vi "GeoData.vi"() -> ()   [LabVIEW 2017] (continued)
Brandywine\tMD\tCharles County\tH1\n20616\t24017\tBryans road\tMD\tCharles County\tH1\n21613\t24019\tCambridge\tMD\tDorchester County\tH1\n21648\t24019\tMadison\tMD\tDorchester County\tH1\n21626\t24019\tCrapo\tMD\tDorchester County\tH1\n21675\t24019\tWingate\tMD\tDorchester County\tH1\n21669\t24019\tTaylors island\tMD\tDorchester County\tH1\n21655\t24019\tPreston\tMD\tDorchester County\tH1\n21664\t24019\tSecretary\tMD\tDorchester County\tH1\n21835\t24019\tLinkwood\tMD\tDorchester County\tH1\n21672\t24019\tToddville\tMD\tDorchester County\tH1\n21622\t24019\tChurch creek\tMD\tDorchester County\tH1\n21631\t24019\tEast new market\tMD\tDorchester County\tH1\n21659\t24019\tRhodesdale\tMD\tDorchester County\tH1\n21632\t24019\tFederalsburg\tMD\tDorchester County\tH1\n21643\t24019\tHurlock\tMD\tDorchester County\tH1\n21677\t24019\tWoolford\tMD\tDorchester County\tH1\n21627\t24019\tCrocheron\tMD\tDorchester County\tH1\n21869\t24019\tVienna\tMD\tDorchester County\tH1\n21634\t24019\tFishing creek\tMD\tDorchester County\tH1\n20842\t24021\tDickerson\tMD\tFrederick County\tH1\n21757\t24021\tKeymar\tMD\tFrederick County\tH1\n21783\t24021\tSmithsburg\tMD\tFrederick County\tH1\n21719\t24021\tCascade\tMD\tFrederick County\tH1\n21759\t24021\tLadiesburg\tMD\tFrederick County\tH1\n21704\t24021\tFrederick\tMD\tFrederick County\tH1\n21771\t24021\tMount airy\tMD\tFrederick County\tH1\n21773\t24021\tMyersville\tMD\tFrederick County\tH1\n21787\t24021\tTaneytown\tMD\tFrederick County\tH1\n21793\t24021\tWalkersville\tMD\tFrederick County\tH1\n21798\t24021\tWoodsboro\tMD\tFrederick County\tH1\n21790\t24021\tTuscarora\tMD\tFrederick County\tH1\n20871\t24021\tClarksburg\tMD\tFrederick County\tH1\n21774\t24021\tNew market\tMD\tFrederick County\tH1\n21727\t24021\tEmmitsburg\tMD\tFrederick County\tH1\n21769\t24021\tMiddletown\tMD\tFrederick County\tH1\n21780\t24021\tSabillasville\tMD\tFrederick County\tH1\n21714\t24021\tBraddock heights\tMD\tFrederick County\tH1\n21703\t24021\tFrederick\tMD\tFrederick County\tH1\n21770\t24021\tMonrovia\tMD\tFrederick County\tH1\n21754\t24021\tIjamsville\tMD\tFrederick County\tH1\n21755\t24021\tJefferson\tMD\tFrederick County\tH1\n21717\t24021\tBuckeystown\tMD\tFrederick County\tH1\n21778\t24021\tRocky ridge\tMD\tFrederick County\tH1\n21776\t24021\tNew windsor\tMD\tFrederick County\tH1\n21791\t24021\tUnion bridge\tMD\tFrederick County\tH1\n21762\t24021\tLibertytown\tMD\tFrederick County\tH1\n21716\t24021\tBrunswick\tMD\tFrederick County\tH1\n21710\t24021\tAdamstown\tMD\tFrederick County\tH1\n21758\t24021\tKnoxville\tMD\tFrederick County\tH1\n21777\t24021\tPoint of rocks\tMD\tFrederick County\tH1\n21775\t24021\tNew midway\tMD\tFrederick County\tH1\n21701\t24021\tFrederick\tMD\tFrederick County\tH1\n21702\t24021\tFrederick\tMD\tFrederick County\tH1\n21713\t24021\tBoonsboro\tMD\tFrederick County\tH1\n21705\t24021\tFrederick\tMD\tFrederick County\tH1\n21788\t24021\tThurmont\tMD\tFrederick County\tH1\n21718\t24021\tBurkittsville\tMD\tFrederick County\tH1\n21531\t24023\tFriendsville\tMD\tGarrett County\tH1\n21538\t24023\tKitzmiller\tMD\tGarrett County\tH1\n21562\t24023\tWesternport\tMD\tGarrett County\tH1\n21536\t24023\tGrantsville\tMD\tGarrett County\tH1\n21521\t24023\tBarton\tMD\tGarrett County\tH1\n21523\t24023\tBloomington\tMD\tGarrett County\tH1\n21532\t24023\tFrostburg\tMD\tGarrett County\tH1\n21541\t24023\tMc henry\tMD\tGarrett County\tH1\n21561\t24023\tSwanton\tMD\tGarrett County\tH1\n21522\t24023\tBittinger\tMD\tGarrett County\tH1\n21539\t24023\tLonaconing\tMD\tGarrett County\tH1\n21520\t24023\tAccident\tMD\tGarrett County\tH1\n21550\t24023\tOakland\tMD\tGarrett County\tH1\n21014\t24025\tBel air\tMD\tHarford County\tH1\n21034\t24025\tDarlington\tMD\tHarford County\tH1\n21050\t24025\tForest hill\tMD\tHarford County\tH1\n21087\t24025\tKingsville\tMD\tHarford County\tH1\n21160\t24025\tWhiteford\tMD\tHarford County\tH1\n21154\t24025\tStreet\tMD\tHarford County\tH1\n21010\t24025\tGunpowder\tMD\tHarford County\tH1\n21047\t24025\tFallston\tMD\tHarford County\tH1\n21084\t24025\tJarrettsville\tMD\tHarford County\tH1\n21078\t24025\tHavre de grace\tMD\tHarford County\tH1\n21018\t24025\tBenson\tMD\tHarford County\tH1\n21001\t24025\tAberdeen\tMD\tHarford County\tH1\n21028\t24025\tChurchville\tMD\tHarford County\tH1\n21085\t24025\tJoppa\tMD\tHarford County\tH1\n21111\t24025\tMonkton\tMD\tHarford County\tH1\n21130\t24025\tPerryman\tMD\tHarford County\tH1\n21005\t24025\tAberdeen proving ground\tMD\tHarford County\tH1\n21082\t24025\tHydes\tMD\tHarford County\tH1\n21132\t24025\tPylesville\tMD\tHarford County\tH1\n21161\t24025\tWhite hall\tMD\tHarford County\tH1\n21017\t24025\tBelcamp\tMD\tHarford County\tH1\n21009\t24025\tAbingdon\tMD\tHarford County\tH1\n21040\t24025\tEdgewood\tMD\tHarford County\tH1\n21015\t24025\tBel air\tMD\tHarford County\tH1\n21013\t24025\tBaldwin\tMD\tHarford County\tH1\n21043\t24027\tEllicott city\tMD\tHoward County\tH1\n21046\t24027\tColumbia\tMD\tHoward County\tH1\n21737\t24027\tGlenelg\tMD\tHoward County\tH1\n20777\t24027\tHighland\tMD\tHoward County\tH1\n21771\t24027\tMount airy\tMD\tHoward County\tH1\n21784\t24027\tSykesville\tMD\tHoward County\tH1\n21738\t24027\tGlenwood\tMD\tHoward County\tH1\n21794\t24027\tWest friendship\tMD\tHoward County\tH1\n20723\t24027\tLaurel\tMD\tHoward County\tH1\n20794\t24027\tJessup\tMD\tHoward County\tH1\n21044\t24027\tColumbia\tMD\tHoward County\tH1\n21041\t24027\tEllicott city\tMD\tHoward County\tH1\n21042\t24027\tEllicott city\tMD\tHoward County\tH1\n21036\t24027\tDayton\tMD\tHoward County\tH1\n21075\t24027\tElkridge\tMD\tHoward County\tH1\n21163\t24027\tWoodstock\tMD\tHoward County\tH1\n21765\t24027\tLisbon\tMD\tHoward County\tH1\n21150\t24027\tSimpsonville\tMD\tHoward County\tH1\n20763\t24027\tSavage\tMD\tHoward County\tH1\n20759\t24027\tFulton\tMD\tHoward County\tH1\n21029\t24027\tClarksville\tMD\tHoward County\tH1\n21076\t24027\tHanover\tMD\tHoward County\tH1\n21723\t24027\tCooksville\tMD\tHoward County\tH1\n20701\t24027\tAnnapolis junction\tMD\tHoward County\tH1\n20833\t24027\tBrookeville\tMD\tHoward County\tH1\n21045\t24027\tColumbia\tMD\tHoward County\tH1\n21797\t24027\tWoodbine\tMD\tHoward County\tH1\n21104\t24027\tMarriottsville\tMD\tHoward County\tH1\n21645\t24029\tKennedyville\tMD\tKent County\tH1\n21667\t24029\tStill pond\tMD\tKent County\tH1\n21610\t24029\tBetterton\tMD\tKent County\tH1\n21635\t24029\tGalena\tMD\tKent County\tH1\n21651\t24029\tMillington\tMD\tKent County\tH1\n21678\t24029\tWorton\tMD\tKent County\tH1\n21690\t24029\tChestertown\tMD\tKent County\tH1\n21930\t24029\tGeorgetown\tMD\tKent County\tH1\n21620\t24029\tChestertown\tMD\tKent County\tH1\n21661\t24029\tRock hall\tMD\tKent County\tH1\n21650\t24029\tMassey\tMD\tKent County\tH1\n20815\t24031\tChevy chase\tMD\tMontgomery County\tH1\n20816\t24031\tBethesda\tMD\tMontgomery County\tH1\n20841\t24031\tBoyds\tMD\tMontgomery County\tH1\n20842\t24031\tDickerson\tMD\tMontgomery County\tH1\n20906\t24031\tSilver spring\tMD\tMontgomery County\tH1\n20777\t24031\tHighland\tMD\tMontgomery County\tH1\n20884\t24031\tGaithersburg\tMD\tMontgomery County\tH1\n20818\t24031\tCabin john\tMD\tMontgomery County\tH1\n20852\t24031\tRockville\tMD\tMontgomery County\tH1\n20914\t24031\tSilver spring\tMD\tMontgomery County\tH1\n20915\t24031\tSilver spring\tMD\tMontgomery County\tH1\n21771\t24031\tMount airy\tMD\tMontgomery County\tH1\n20880\t24031\tWashington grove\tMD\tMontgomery County\tH1\n20918\t24031\tSilver spring\tMD\tMontgomery County\tH1\n20849\t24031\tRockville\tMD\tMontgomery County\tH1\n20911\t24031\tSilver spring\tMD\tMontgomery County\tH1\n20859\t24031\tPotomac\tMD\tMontgomery County\tH1\n20993\t24031\tSilver spring\tMD\tMontgomery County\tH1\n20854\t24031\tPotomac\tMD\tMontgomery County\tH1\n20868\t24031\tSpencerville\tMD\tMontgomery County\tH1\n20871\t24031\tClarksburg\tMD\tMontgomery County\tH1\n20882\t24031\tGaithersburg\tMD\tMontgomery County\tH1\n20838\t24031\tBarnesville\tMD\tMontgomery County\tH1\n20898\t24031\tGaithersburg\tMD\tMontgomery County\tH1\n20830\t24031\tOlney\tMD\tMontgomery County\tH1\n20892\t24031\tBethesda\tMD\tMontgomery County\tH1\n20783\t24031\tHyattsville\tMD\tMontgomery County\tH1\n20832\t24031\tOlney\tMD\tMontgomery County\tH1\n20861\t24031\tAshton\tMD\tMontgomery County\tH1\n20903\t24031\tSilver spring\tMD\tMontgomery County\tH1\n21770\t24031\tMonrovia\tMD\tMontgomery County\tH1\n20862\t24031\tBrinklow\tMD\tMontgomery County\tH1\n20811\t24031\tBethesda\tMD\tMontgomery County\tH1\n20817\t24031\tBethesda\tMD\tMontgomery County\tH1\n20874\t24031\tGermantown\tMD\tMontgomery County\tH1\n20851\t24031\tRockville\tMD\tMontgomery County\tH1\n20860\t24031\tSandy spring\tMD\tMontgomery County\tH1\n20901\t24031\tSilver spring\tMD\tMontgomery County\tH1\n20902\t24031\tSilver spring\tMD\tMontgomery County\tH1\n20899\t24031\tGaithersburg\tMD\tMontgomery County\tH1\n20827\t24031\tBethesda\tMD\tMontgomery County\tH1\n20812\t24031\tGlen echo\tMD\tMontgomery County\tH1\n20847\t24031\tRockville\tMD\tMontgomery County\tH1\n20839\t24031\tBeallsville\tMD\tMontgomery County\tH1\n20857\t24031\tRockville\tMD\tMontgomery County\tH1\n20058\t24031\tWashington\tMD\tMontgomery County\tH1\n20707\t24031\tLaurel\tMD\tMontgomery County\tH1\n20787\t24031\tHyattsville\tMD\tMontgomery County\tH1\n20853\t24031\tRockville\tMD\tMontgomery County\tH1\n20855\t24031\tDerwood\tMD\tMontgomery County\tH1\n20872\t24031\tDamascus\tMD\tMontgomery County\tH1\n20875\t24031\tGermantown\tMD\tMontgomery County\tH1\n20878\t24031\tGaithersburg\tMD\tMontgomery County\tH1\n20886\t24031\tMontgomery village\tMD\tMontgomery County\tH1\n20891\t24031\tKensington\tMD\tMontgomery County\tH1\n20912\t24031\tTakoma park\tMD\tMontgomery County\tH1\n20824\t24031\tBethesda\tMD\tMontgomery County\tH1\n20885\t24031\tGaithersburg\tMD\tMontgomery County\tH1\n20907\t24031\tSilver spring\tMD\tMontgomery County\tH1\n20825\t24031\tChevy chase\tMD\tMontgomery County\tH1\n20883\t24031\tGaithersburg\tMD\tMontgomery County\tH1\n20894\t24031\tBethesda\tMD\tMontgomery County\tH1\n20837\t24031\tPoolesville\tMD\tMontgomery County\tH1\n20904\t24031\tSilver spring\tMD\tMontgomery County\tH1\n20895\t24031\tKensington\tMD\tMontgomery County\tH1\n20879\t24031\tGaithersburg\tMD\tMontgomery County\tH1\n20877\t24031\tGaithersburg\tMD\tMontgomery County\tH1\n20910\t24031\tSilver spring\tMD\tMontgomery County\tH1\n20913\t24031\tTakoma park\tMD\tMontgomery County\tH1\n20848\t24031\tRockville\tMD\tMontgomery County\tH1\n20896\t24031\tGarrett park\tMD\tMontgomery County\tH1\n20889\t24031\tBethesda\tMD\tMontgomery County\tH1\n20916\t24031\tSilver spring\tMD\tMontgomery County\tH1\n20810\t24031\tBethesda\tMD\tMontgomery County\tH1\n20814\t24031\tBethesda\tMD\tMontgomery County\tH1\n20850\t24031\tRockville\tMD\tMontgomery County\tH1\n20833\t24031\tBrookeville\tMD\tMontgomery County\tH1\n20876\t24031\tGermantown\tMD\tMontgomery County\tH1\n20866\t24031\tBurtonsville\tMD\tMontgomery County\tH1\n20905\t24031\tSilver spring\tMD\tMontgomery County\tH1\n21797\t24031\tWoodbine\tMD\tMontgomery County\tH1\n20207\t24031\tWashington\tMD\tMontgomery County\tH1\n20705\t24033\tBeltsville\tMD\tPrince George's County\tH1\n20710\t24033\tBladensburg\tMD\tPrince George's County\tH1\n20721\t24033\tBowie\tMD\tPrince George's County\tH1\n20623\t24033\tCheltenham\tMD\tPrince George's County\tH1\n20718\t24033\tBowie\tMD\tPrince George's County\tH1\n20773\t24033\tUpper marlboro\tMD\tPrince George's County\tH1\n20799\t24033\tCapitol heights\tMD\tPrince George's County\tH1\n20720\t24033\tBowie\tMD\tPrince George's County\tH1\n20715\t24033\tBowie\tMD\tPrince George's County\tH1\n20726\t24033\tLaurel\tMD\tPrince George's County\tH1\n20742\t24033\tCollege park\tMD\tPrince George's County\tH1\n20771\t24033\tGreenbelt\tMD\tPrince George's County\tH1\n20782\t24033\tHyattsville\tMD\tPrince George's County\tH1\n20791\t24033\tCapitol heights\tMD\tPrince George's County\tH1\n20775\t24033\tUpper marlboro\tMD\tPrince George's County\tH1\n20757\t24033\tTemple hills\tMD\tPrince George's County\tH1\n20749\t24033\tFort washington\tMD\tPrince George's County\tH1\n20750\t24033\tOxon hill\tMD\tPrince George's County\tH1\n20389\t24033\tWashington\tMD\tPrince George's County\tH1\n20395\t24033\tWashington\tMD\tPrince George's County\tH1\n20716\t24033\tBowie\tMD\tPrince George's County\tH1\n20724\t24033\tLaurel\tMD\tPrince George's County\tH1\n20745\t24033\tOxon hill\tMD\tPrince George's County\tH1\n20769\t24033\tGlenn dale\tMD\tPrince George's County\tH1\n20772\t24033\tUpper marlboro\tMD\tPrince George's County\tH1\n20783\t24033\tHyattsville\tMD\tPrince George's County\tH1\n20903\t24033\tSilver spring\tMD\tPrince George's County\tH1\n20709\t24033\tLaurel\tMD\tPrince George's County\tH1\n20741\t24033\tCollege park\tMD\tPrince George's County\tH1\n20768\t24033\tGreenbelt\tMD\tPrince George's County\tH1\n20703\t24033\tLanham\tMD\tPrince George's County\tH1\n20731\t24033\tCapitol heights\tMD\tPrince George's County\tH1\n20608\t24033\tAquasco\tMD\tPrince George's County\tH1\n20708\t24033\tLaurel\tMD\tPrince George's County\tH1\n20712\t24033\tMount rainier\tMD\tPrince George's County\tH1\n20740\t24033\tCollege park\tMD\tPrince George's County\tH1\n20792\t24033\tUpper marlboro\tMD\tPrince George's County\tH1\n20753\t24033\tDistrict heights\tMD\tPrince George's County\tH1\n20707\t24033\tLaurel\tMD\tPrince George's County\tH1\n20706\t24033\tLanham\tMD\tPrince George's County\tH1\n20743\t24033\tCapitol heights\tMD\tPrince George's County\tH1\n20737\t24033\tRiverdale\tMD\tPrince George's County\tH1\n20748\t24033\tTemple hills\tMD\tPrince George's County\tH1\n20774\t24033\tUpper marlboro\tMD\tPrince George's County\tH1\n20784\t24033\tHyattsville\tMD\tPrince George's County\tH1\n20912\t24033\tTakoma park\tMD\tPrince George's County\tH1\n20599\t24033\tWashington\tMD\tPrince George's County\tH1\n20601\t24033\tWaldorf\tMD\tPrince George's County\tH1\n20735\t24033\tClinton\tMD\tPrince George's County\tH1\n20746\t24033\tSuitland\tMD\tPrince George's County\tH1\n20781\t24033\tHyattsville\tMD\tPrince George's County\tH1\n20904\t24033\tSilver spring\tMD\tPrince George's County\tH1\n20725\t24033\tLaurel\tMD\tPrince George's County\tH1\n20722\t24033\tBrentwood\tMD\tPrince George's County\tH1\n20704\t24033\tBeltsville\tMD\tPrince George's County\tH1\n20717\t24033\tBowie\tMD\tPrince George's County\tH1\n20588\t24033\tDhs\tMD\tPrince George's County\tH1\n20790\t24033\tCapitol heights\tMD\tPrince George's County\tH1\n20607\t24033\tAccokeek\tMD\tPrince George's County\tH1\n20613\t24033\tBrandywine\tMD\tPrince George's County\tH1\n20616\t24033\tBryans road\tMD\tPrince George's County\tH1\n20744\t24033\tFort washington\tMD\tPrince George's County\tH1\n20770\t24033\tGreenbelt\tMD\tPrince George's County\tH1\n20747\t24033\tDistrict heights\tMD\tPrince George's County\tH1\n20762\t24033\tAndrews air force base\tMD\tPrince George's County\tH1\n20785\t24033\tHyattsville\tMD\tPrince George's County\tH1\n20866\t24033\tBurtonsville\tMD\tPrince George's County\tH1\n20738\t24033\tRiverdale\tMD\tPrince George's County\tH1\n20233\t24033\tWashington\tMD\tPrince George's County\tH1\n20752\t24033\tSuitland\tMD\tPrince George's County\tH1\n21619\t24035\tChester\tMD\tQueen Anne's County\tH1\n21644\t24035\tIngleside\tMD\tQueen Anne's County\tH1\n21679\t24035\tWye mills\tMD\tQueen Anne's County\tH1\n21656\t24035\tPrice\tMD\tQueen Anne's County\tH1\n21651\t24035\tMillington\tMD\tQueen Anne's County\tH1\n21668\t24035\tSudlersville\tMD\tQueen Anne's County\tH1\n21640\t24035\tHenderson\tMD\tQueen Anne's County\tH1\n21649\t24035\tMarydel\tMD\tQueen Anne's County\tH1\n21638\t24035\tGrasonville\tMD\tQueen Anne's County\tH1\n21657\t24035\tQueen anne\tMD\tQueen Anne's County\tH1\n21666\t24035\tStevensville\tMD\tQueen Anne's County\tH1\n21607\t24035\tBarclay\tMD\tQueen Anne's County\tH1\n21623\t24035\tChurch hill\tMD\tQueen Anne's County\tH1\n21628\t24035\tCrumpton\tMD\tQueen Anne's County\tH1\n21670\t24035\tTempleville\tMD\tQueen Anne's County\tH1\n21620\t24035\tChestertown\tMD\tQueen Anne's County\tH1\n21617\t24035\tCentreville\tMD\tQueen Anne's County\tH1\n21658\t24035\tQueenstown\tMD\tQueen Anne's County\tH1\n20634\t24037\tGreat mills\tMD\tSt. Mary's County\tH1\n20692\t24037\tValley lee\tMD\tSt. Mary's County\tH1\n20626\t24037\tColtons point\tMD\tSt. Mary's County\tH1\n20620\t24037\tCallaway\tMD\tSt. Mary's County\tH1\n20670\t24037\tPatuxent river\tMD\tSt. Mary's County\tH1\n20659\t24037\tMechanicsville\tMD\tSt. Mary's County\tH1\n20630\t24037\tDrayden\tMD\tSt. Mary's County\tH1\n20609\t24037\tAvenue\tMD\tSt. Mary's County\tH1\n20628\t24037\tDameron\tMD\tSt. Mary's County\tH1\n20635\t24037\tHelen\tMD\tSt. Mary's County\tH1\n20622\t24037\tCharlotte hall\tMD\tSt. Mary's County\tH1\n20684\t24037\tSaint inigoes\tMD\tSt. Mary's County\tH1\n20618\t24037\tBushwood\tMD\tSt. Mary's County\tH1\n20686\t24037\tSaint marys city\tMD\tSt. Mary's County\tH1\n20619\t24037\tCalifornia\tMD\tSt. Mary's County\tH1\n20653\t24037\tLexington park\tMD\tSt. Mary's County\tH1\n20690\t24037\tTall timbers\tMD\tSt. Mary's County\tH1\n20660\t24037\tMorganza\tMD\tSt. Mary's County\tH1\n20624\t24037\tClements\tMD\tSt. Mary's County\tH1\n20674\t24037\tPiney point\tMD\tSt. Mary's County\tH1\n20680\t24037\tRidge\tMD\tSt. Mary's County\tH1\n20650\t24037\tLeonardtown\tMD\tSt. Mary's County\tH1\n20606\t24037\tAbell\tMD\tSt. Mary's County\tH1\n20656\t24037\tLoveville\tMD\tSt. Mary's County\tH1\n20687\t24037\tScotland\tMD\tSt. Mary's County\tH1\n20621\t24037\tChaptico\tMD\tSt. Mary's County\tH1\n20636\t24037\tHollywood\tMD\tSt. Mary's County\tH1\n20667\t24037\tPark hall\tMD\tSt. Mary's County\tH1\n20627\t24037\tCompton\tMD\tSt. Mary's County\tH1\n21817\t24039\tCrisfield\tMD\tSomerset County\tH1\n21821\t24039\tDeal island\tMD\tSomerset County\tH1\n21838\t24039\tMarion station\tMD\tSomerset County\tH1\n21851\t24039\tPocomoke city\tMD\tSomerset County\tH1\n21857\t24039\tRehobeth\tMD\tSomerset County\tH1\n21836\t24039\tManokin\tMD\tSomerset County\tH1\n21824\t24039\tEwell\tMD\tSomerset County\tH1\n21866\t24039\tTylerton\tMD\tSomerset County\tH1\n21867\t24039\tUpper fairmount\tMD\tSomerset County\tH1\n21871\t24039\tWestover\tMD\tSomerset County\tH1\n21890\t24039\tWestover\tMD\tSomerset County\tH1\n21853\t24039\tPrincess anne\tMD\tSomerset County\tH1\n21822\t24039\tEden\tMD\tSomerset County\tH1\n21601\t24041\tEaston\tMD\tTalbot County\tH1\n21665\t24041\tSherwood\tMD\tTalbot County\tH1\n21679\t24041\tWye mills\tMD\tTalbot County\tH1\n21671\t24041\tTilghman\tMD\tTalbot County\tH1\n21647\t24041\tMcdaniel\tMD\tTalbot County\tH1\n21657\t24041\tQueen anne\tMD\tTalbot County\tH1\n21673\t24041\tTrappe\tMD\tTalbot County\tH1\n21663\t24041\tSaint michaels\tMD\tTalbot County\tH1\n21652\t24041\tNeavitt\tMD\tTalbot County\tH1\n21654\t24041\tOxford\tMD\tTalbot County\tH1\n21624\t24041\tClaiborne\tMD\tTalbot County\tH1\n21662\t24041\tRoyal oak\tMD\tTalbot County\tH1\n21625\t24041\tCordova\tMD\tTalbot County\tH1\n21676\t24041\tWittman\tMD\tTalbot County\tH1\n21612\t24041\tBozman\tMD\tTalbot County\tH1\n21653\t24041\tNewcomb\tMD\tTalbot County\tH1\n21783\t24043\tSmithsburg\tMD\tWashington County\tH1\n21719\t24043\tCascade\tMD\tWashington County\tH1\n21779\t24043\tRohrersville\tMD\tWashington County\tH1\n21721\t24043\tChewsville\tMD\tWashington County\tH1\n21767\t24043\tMaugansville\tMD\tWashington County\tH1\n21746\t24043\tHagerstown\tMD\tWashington County\tH1\n21781\t24043\tSaint james\tMD\tWashington County\tH1\n21769\t24043\tMiddletown\tMD\tWashington County\tH1\n21780\t24043\tSabillasville\tMD\tWashington County\tH1\n21715\t24043\tBrownsville\tMD\tWashington County\tH1\n21740\t24043\tHagerstown\tMD\tWashington County\tH1\n21755\t24043\tJefferson\tMD\tWashington County\tH1\n21720\t24043\tCavetown\tMD\tWashington County\tH1\n21711\t24043\tBig pool\tMD\tWashington County\tH1\n21750\t24043\tHancock\tMD\tWashington County\tH1\n21733\t24043\tFairplay\tMD\tWashington County\tH1\n21758\t24043\tKnoxville\tMD\tWashington County\tH1\n21795\t24043\tWilliamsport\tMD\tWashington County\tH1\n21756\t24043\tKeedysville\tMD\tWashington County\tH1\n21734\t24043\tFunkstown\tMD\tWashington County\tH1\n21713\t24043\tBoonsboro\tMD\tWashington County\tH1\n21742\t24043\tHagerstown\tMD\tWashington County\tH1\n21741\t24043\tHagerstown\tMD\tWashington County\tH1\n21722\t24043\tClear spring\tMD\tWashington County\tH1\n21782\t24043\tSharpsburg\tMD\tWashington County\tH1\n21802\t24045\tSalisbury\tMD\tWicomico County\tH1\n21875\t24045\tDelmar\tMD\tWicomico County\tH1\n21850\t24045\tPittsville\tMD\tWicomico County\tH1\n21837\t24045\tMardela springs\tMD\tWicomico County\tH1\n21856\t24045\tQuantico\tMD\tWicomico County\tH1\n21852\t24045\tPowellville\tMD\tWicomico County\tH1\n21801\t24045\tSalisbury\tMD\tWicomico County\tH1\n21810\t24045\tAllen\tMD\tWicomico County\tH1\n21874\t24045\tWillards\tMD\tWicomico County\tH1\n21814\t24045\tBivalve\tMD\tWicomico County\tH1\n21830\t24045\tHebron\tMD\tWicomico County\tH1\n21803\t24045\tSalisbury\tMD\tWicomico County\tH1\n21826\t24045\tFruitland\tMD\tWicomico County\tH1\n21840\t24045\tNanticoke\tMD\tWicomico County\tH1\n21861\t24045\tSharptown\tMD\tWicomico County\tH1\n21804\t24045\tSalisbury\tMD\tWicomico County\tH1\n21865\t24045\tTyaskin\tMD\tWicomico County\tH1\n21849\t24045\tParsonsburg\tMD\tWicomico County\tH1\n21822\t24045\tEden\tMD\tWicomico County\tH1\n21872\t24047\tWhaleyville\tMD\tWorcester County\tH1\n21851\t24047\tPocomoke city\tMD\tWorcester County\tH1\n21843\t24047\tOcean city\tMD\tWorcester County\tH1\n21863\t24047\tSnow hill\tMD\tWorcester County\tH1\n21841\t24047\tNewark\tMD\tWorcester County\tH1\n21792\t24047\tUnionville\tMD\tWorcester County\tH1\n21842\t24047\tOcean city\tMD\tWorcester County\tH1\n21864\t24047\tStockton\tMD\tWorcester County\tH1\n21862\t24047\tShowell\tMD\tWorcester County\tH1\n21804\t24047\tSalisbury\tMD\tWorcester County\tH1\n21811\t24047\tBerlin\tMD\tWorcester County\tH1\n21829\t24047\tGirdletree\tMD\tWorcester County\tH1\n21813\t24047\tBishopville\tMD\tWorcester County\tH1\n21822\t24047\tEden\tMD\tWorcester County\tH1\n21202\t24510\tBaltimore\tMD\tBaltimore city\tC7\n21205\t24510\tBaltimore\tMD\tBaltimore city\tC7\n21207\t24510\tGwynn oak\tMD\tBaltimore city\tC7\n21214\t24510\tBaltimore\tMD\tBaltimore city\tC7\n21210\t24510\tBaltimore\tMD\tBaltimore city\tC7\n21218\t24510\tBaltimore\tMD\tBaltimore city\tC7\n21223\t24510\tBaltimore\tMD\tBaltimore city\tC7\n21237\t24510\tRosedale\tMD\tBaltimore city\tC7\n21234\t24510\tParkville\tMD\tBaltimore city\tC7\n21236\t24510\tNottingham\tMD\tBaltimore city\tC7\n21233\t24510\tBaltimore\tMD\tBaltimore city\tC7\n21263\t24510\tBaltimore\tMD\tBaltimore city\tC7\n21216\t24510\tBaltimore\tMD\tBaltimore city\tC7\n21278\t24510\tBaltimore\tMD\tBaltimore city\tC7\n21206\t24510\tBaltimore\tMD\tBaltimore city\tC7\n21217\t24510\tBaltimore\tMD\tBaltimore city\tC7\n21222\t24510\tDundalk\tMD\tBaltimore city\tC7\n21228\t24510\tCatonsville\tMD\tBaltimore city\tC7\n21229\t24510\tBaltimore\tMD\tBaltimore city\tC7\n21290\t24510\tBaltimore\tMD\tBaltimore city\tC7\n21209\t24510\tBaltimore\tMD\tBaltimore city\tC7\n21212\t24510\tBaltimore\tMD\tBaltimore city\tC7\n21226\t24510\tCurtis bay\tMD\tBaltimore city\tC7\n21208\t24510\tPikesville\tMD\tBaltimore city\tC7\n21203\t24510\tBaltimore\tMD\tBaltimore city\tC7\n21270\t24510\tBaltimore\tMD\tBaltimore city\tC7\n21213\t24510\tBaltimore\tMD\tBaltimore city\tC7\n21215\t24510\tBaltimore\tMD\tBaltimore city\tC7\n21224\t24510\tBaltimore\tMD\tBaltimore city\tC7\n21230\t24510\tBaltimore\tMD\tBaltimore city\tC7\n21227\t24510\tHalethorpe\tMD\tBaltimore city\tC7\n21239\t24510\tBaltimore\tMD\tBaltimore city\tC7\n21287\t24510\tBaltimore\tMD\tBaltimore city\tC7\n21201\t24510\tBaltimore\tMD\tBaltimore city\tC7\n21211\t24510\tBaltimore\tMD\tBaltimore city\tC7\n21225\t24510\tBrooklyn\tMD\tBaltimore city\tC7\n21231\t24510\tBaltimore\tMD\tBaltimore city\tC7\n21281\t24510\tBaltimore\tMD\tBaltimore city\tC7\n21251\t24510\tBaltimore\tMD\tBaltimore city\tC7\n2642\t25001\tEastham\tMA\tBarnstable County\tH1\n2645\t25001\tHarwich\tMA\tBarnstable County\tH1\n2660\t25001\tSouth dennis\tMA\tBarnstable County\tH1\n2657\t25001\tProvincetown\tMA\tBarnstable County\tH1\n2659\t25001\tSouth chatham\tMA\tBarnstable County\tH1\n2669\t25001\tWest chatham\tMA\tBarnstable County\tH1\n2534\t25001\tCataumet\tMA\tBarnstable County\tH1\n2634\t25001\tCenterville\tMA\tBarnstable County\tH1\n2540\t25001\tFalmouth\tMA\tBarnstable County\tH1\n2553\t25001\tMonument beach\tMA\tBarnstable County\tH1\n2542\t25001\tBuzzards bay\tMA\tBarnstable County\tH1\n2601\t25001\tHyannis\tMA\tBarnstable County\tH1\n2648\t25001\tMarstons mills\tMA\tBarnstable County\tH1\n2647\t25001\tHyannis port\tMA\tBarnstable County\tH1\n2644\t25001\tForestdale\tMA\tBarnstable County\tH1\n2543\t25001\tWoods hole\tMA\tBarnstable County\tH1\n2631\t25001\tBrewster\tMA\tBarnstable County\tH1\n2649\t25001\tMashpee\tMA\tBarnstable County\tH1\n2653\t25001\tOrleans\tMA\tBarnstable County\tH1\n2668\t25001\tWest barnstable\tMA\tBarnstable County\tH1\n2650\t25001\tNorth chatham\tMA\tBarnstable County\tH1\n2672\t25001\tWest hyannisport\tMA\tBarnstable County\tH1\n2561\t25001\tSagamore\tMA\tBarnstable County\tH1\n2652\t25001\tNorth truro\tMA\tBarnstable County\tH1\n2532\t25001\tBuzzards bay\tMA\tBarnstable County\tH1\n2536\t25001\tEast falmouth\tMA\tBarnstable County\tH1\n2633\t25001\tChatham\tMA\tBarnstable County\tH1\n2661\t25001\tSouth harwich\tMA\tBarnstable County\tH1\n2666\t25001\tTruro\tMA\tBarnstable County\tH1\n2643\t25001\tEast orleans\tMA\tBarnstable County\tH1\n2559\t25001\tPocasset\tMA\tBarnstable County\tH1\n2664\t25001\tSouth yarmouth\tMA\tBarnstable County\tH1\n2670\t25001\tWest dennis\tMA\tBarnstable County\tH1\n2556\t25001\tNorth falmouth\tMA\tBarnstable County\tH1\n2360\t25001\tPlymouth\tMA\tBarnstable County\tH1\n2563\t25001\tSandwich\tMA\tBarnstable County\tH1\n2632\t25001\tCenterville\tMA\tBarnstable County\tH1\n2646\t25001\tHarwich port\tMA\tBarnstable County\tH1\n2675\t25001\tYarmouth port\tMA\tBarnstable County\tH1\n2655\t25001\tOsterville\tMA\tBarnstable County\tH1\n2637\t25001\tCummaquid\tMA\tBarnstable County\tH1\n2663\t25001\tSouth wellfleet\tMA\tBarnstable County\tH1\n2537\t25001\tEast sandwich\tMA\tBarnstable County\tH1\n2630\t25001\tBarnstable\tMA\tBarnstable County\tH1\n2574\t25001\tWest falmouth\tMA\tBarnstable County\tH1\n2639\t25001\tDennis port\tMA\tBarnstable County\tH1\n2662\t25001\tSouth orleans\tMA\tBarnstable County\tH1\n2651\t25001\tNorth eastham\tMA\tBarnstable County\tH1\n2562\t25001\tSagamore beach\tMA\tBarnstable County\tH1\n2638\t25001\tDennis\tMA\tBarnstable County\tH1\n2635\t25001\tCotuit\tMA\tBarnstable County\tH1\n2667\t25001\tWellfleet\tMA\tBarnstable County\tH1\n2673\t25001\tWest yarmouth\tMA\tBarnstable County\tH1\n2671\t25001\tWest harwich\tMA\tBarnstable County\tH1\n2541\t25001\tFalmouth\tMA\tBarnstable County\tH1\n2641\t25001\tEast dennis\tMA\tBarnstable County\tH1\n1026\t25003\tCummington\tMA\tBerkshire County\tH4\n1220\t25003\tAdams\tMA\tBerkshire County\tH4\n1270\t25003\tWindsor\tMA\tBerkshire County\tH4\n1260\t25003\tSouth lee\tMA\tBerkshire County\tH4\n1263\t25003\tStockbridge\tMA\tBerkshire County\tH4\n1235\t25003\tHinsdale\tMA\tBerkshire County\tH4\n1029\t25003\tEast otis\tMA\tBerkshire County\tH4\n1242\t25003\tLenox dale\tMA\tBerkshire County\tH4\n1237\t25003\tLanesborough\tMA\tBerkshire County\tH4\n1257\t25003\tSheffield\tMA\tBerkshire County\tH4\n1262\t25003\tStockbridge\tMA\tBerkshire County\tH4\n1266\t25003\tWest stockbridge\tMA\tBerkshire County\tH4\n1258\t25003\tSouth egremont\tMA\tBerkshire County\tH4\n1244\t25003\tMill river\tMA\tBerkshire County\tH4\n1225\t25003\tCheshire\tMA\tBerkshire County\tH4\n1240\t25003\tLenox\tMA\tBerkshire County\tH4\n1255\t25003\tSandisfield\tMA\tBerkshire County\tH4\n1222\t25003\tAshley falls\tMA\tBerkshire County\tH4\n1202\t25003\tPittsfield\tMA\tBerkshire County\tH4\n1253\t25003\tOtis\tMA\tBerkshire County\tH4\n1229\t25003\tGlendale\tMA\tBerkshire County\tH4\n1252\t25003\tNorth egremont\tMA\tBerkshire County\tH4\n1201\t25003\tPittsfield\tMA\tBerkshire County\tH4\n1247\t25003\tNorth adams\tMA\tBerkshire County\tH4\n1223\t25003\tBecket\tMA\tBerkshire County\tH4\n1230\t25003\tGreat barrington\tMA\tBerkshire County\tH4\n1070\t25003\tPlainfield\tMA\tBerkshire County\tH4\n1254\t25003\tRichmond\tMA\tBerkshire County\tH4\n1226\t25003\tDalton\tMA\tBerkshire County\tH4\n1008\t25003\tBlandford\tMA\tBerkshire County\tH4\n1236\t25003\tHousatonic\tMA\tBerkshire County\tH4\n1011\t25003\tChester\tMA\tBerkshire County\tH4\n1259\t25003\tSouthfield\tMA\tBerkshire County\tH4\n1256\t25003\tSavoy\tMA\tBerkshire County\tH4\n1238\t25003\tLee\tMA\tBerkshire County\tH4\n1227\t25003\tDalton\tMA\tBerkshire County\tH4\n1224\t25003\tBerkshire\tMA\tBerkshire County\tH4\n1267\t25003\tWilliamstown\tMA\tBerkshire County\tH4\n1367\t25003\tRowe\tMA\tBerkshire County\tH4\n1343\t25003\tDrury\tMA\tBerkshire County\tH4\n1245\t25003\tMonterey\tMA\tBerkshire County\tH4\n1264\t25003\tTyringham\tMA\tBerkshire County\tH4\n2762\t25005\tPlainville\tMA\tBristol County\tH1\n2770\t25005\tRochester\tMA\tBristol County\tH1\n2771\t25005\tSeekonk\tMA\tBristol County\tH1\n2790\t25005\tWestport\tMA\tBristol County\tH1\n2768\t25005\tRaynham center\tMA\tBristol County\tH1\n2324\t25005\tBridgewater\tMA\tBristol County\tH1\n2724\t25005\tFall river\tMA\tBristol County\tH1\n2702\t25005\tAssonet\tMA\tBristol County\tH1\n2745\t25005\tNew bedford\tMA\tBristol County\tH1\n2760\t25005\tNorth attleboro\tMA\tBristol County\tH1\n2766\t25005\tNorton\tMA\tBristol County\tH1\n2763\t25005\tAttleboro falls\tMA\tBristol County\tH1\n2347\t25005\tLakeville\tMA\tBristol County\tH1\n2568\t25005\tVineyard haven\tMA\tBristol County\tH1\n2725\t25005\tSomerset\tMA\tBristol County\tH1\n2723\t25005\tFall river\tMA\tBristol County\tH1\n2740\t25005\tNew bedford\tMA\tBristol County\tH1\n2741\t25005\tNew bedford\tMA\tBristol County\tH1\n2721\t25005\tFall river\tMA\tBristol County\tH1\n2718\t25005\tEast taunton\tMA\tBristol County\tH1\n2764\t25005\tNorth dighton\tMA\tBristol County\tH1\n2746\t25005\tNew bedford\tMA\tBristol County\tH1\n2357\t25005\tNorth easton\tMA\tBristol County\tH1\n2048\t25005\tMansfield\tMA\tBristol County\tH1\n2715\t25005\tDighton\tMA\tBristol County\tH1\n2748\t25005\tSouth dartmouth\tMA\tBristol County\tH1\n2780\t25005\tTaunton\tMA\tBristol County\tH1\n2334\t25005\tEaston\tMA\tBristol County\tH1\n2779\t25005\tBerkley\tMA\tBristol County\tH1\n2712\t25005\tChartley\tMA\tBristol County\tH1\n2742\t25005\tNew bedford\tMA\tBristol County\tH1\n2743\t25005\tAcushnet\tMA\tBristol County\tH1\n2767\t25005\tRaynham\tMA\tBristol County\tH1\n2722\t25005\tFall river\tMA\tBristol County\tH1\n2356\t25005\tNorth easton\tMA\tBristol County\tH1\n2375\t25005\tSouth easton\tMA\tBristol County\tH1\n2703\t25005\tAttleboro\tMA\tBristol County\tH1\n2720\t25005\tFall river\tMA\tBristol County\tH1\n2717\t25005\tEast freetown\tMA\tBristol County\tH1\n2726\t25005\tSomerset\tMA\tBristol County\tH1\n2777\t25005\tSwansea\tMA\tBristol County\tH1\n2791\t25005\tWestport point\tMA\tBristol County\tH1\n2719\t25005\tFairhaven\tMA\tBristol County\tH1\n2747\t25005\tNorth dartmouth\tMA\tBristol County\tH1\n2744\t25005\tNew bedford\tMA\tBristol County\tH1\n2769\t25005\tRehoboth\tMA\tBristol County\tH1\n2761\t25005\tNorth attleboro\tMA\tBristol County\tH1\n2535\t25007\tChilmark\tMA\tDukes County\tH1\n2539\t25007\tEdgartown\tMA\tDukes County\tH1\n2575\t25007\tWest tisbury\tMA\tDukes County\tH1\n2568\t25007\tVineyard haven\tMA\tDukes County\tH1\n2713\t25007\tCuttyhunk\tMA\tDukes County\tH1\n2552\t25007\tMenemsha\tMA\tDukes County\tH1\n2557\t25007\tOak bluffs\tMA\tDukes County\tH1\n1810\t25009\tAndover\tMA\tEssex County\tH4\n1902\t25009\tLynn\tMA\tEssex County\tH4\n1960\t25009\tPeabody\tMA\tEssex County\tH4\n1970\t25009\tSalem\tMA\tEssex County\tH4\n1982\t25009\tSouth hamilton\tMA\tEssex County\tH4\n1985\t25009\tWest newbury\tMA\tEssex County\tH4\n1842\t25009\tLawrence\tMA\tEssex County\tH4\n1936\t25009\tHamilton\tMA\tEssex County\tH4\n1812\t25009\tAndover\tMA\tEssex County\tH4\n1876\t25009\tTewksbury\tMA\tEssex County\tH4\n1880\t25009\tWakefield\tMA\tEssex County\tH4\n1915\t25009\tBeverly\tMA\tEssex County\tH4\n1952\t25009\tSalisbury\tMA\tEssex County\tH4\n1835\t25009\tHaverhill\tMA\tEssex County\tH4\n1901\t25009\tLynn\tMA\tEssex County\tH4\n1929\t25009\tEssex\tMA\tEssex County\tH4\n1984\t25009\tWenham\tMA\tEssex County\tH4\n1961\t25009\tPeabody\tMA\tEssex County\tH4\n5501\t25009\tAndover\tMA\tEssex County\tH4\n1910\t25009\tLynn\tMA\tEssex County\tH4\n1834\t25009\tGroveland\tMA\tEssex County\tH4\n1841\t25009\tLawrence\tMA\tEssex County\tH4\n1844\t25009\tMethuen\tMA\tEssex County\tH4\n1904\t25009\tLynn\tMA\tEssex County\tH4\n1922\t25009\tByfield\tMA\tEssex County\tH4\n1965\t25009\tPrides crossing\tMA\tEssex County\tH4\n1899\t25009\tAndover\tMA\tEssex County\tH4\n1833\t25009\tGeorgetown\tMA\tEssex County\tH4\n1913\t25009\tAmesbury\tMA\tEssex County\tH4\n1930\t25009\tGloucester\tMA\tEssex County\tH4\n1938\t25009\tIpswich\tMA\tEssex County\tH4\n1969\t25009\tRowley\tMA\tEssex County\tH4\n1937\t25009\tHathorne\tMA\tEssex County\tH4\n1826\t25009\tDracut\tMA\tEssex County\tH4\n1832\t25009\tHaverhill\tMA\tEssex County\tH4\n1843\t25009\tLawrence\tMA\tEssex County\tH4\n1908\t25009\tNahant\tMA\tEssex County\tH4\n1831\t25009\tHaverhill\tMA\tEssex County\tH4\n1971\t25009\tSalem\tMA\tEssex County\tH4\n1885\t25009\tWest boxford\tMA\tEssex County\tH4\n1830\t25009\tHaverhill\tMA\tEssex County\tH4\n1840\t25009\tLawrence\tMA\tEssex County\tH4\n1860\t25009\tMerrimac\tMA\tEssex County\tH4\n1905\t25009\tLynn\tMA\tEssex County\tH4\n1903\t25009\tLynn\tMA\tEssex County\tH4\n1907\t25009\tSwampscott\tMA\tEssex County\tH4\n1940\t25009\tLynnfield\tMA\tEssex County\tH4\n1945\t25009\tMarblehead\tMA\tEssex County\tH4\n1951\t25009\tNewbury\tMA\tEssex County\tH4\n1966\t25009\tRockport\tMA\tEssex County\tH4\n1931\t25009\tGloucester\tMA\tEssex County\tH4\n1845\t25009\tNorth andover\tMA\tEssex County\tH4\n1906\t25009\tSaugus\tMA\tEssex County\tH4\n1921\t25009\tBoxford\tMA\tEssex County\tH4\n1923\t25009\tDanvers\tMA\tEssex County\tH4\n1944\t25009\tManchester\tMA\tEssex County\tH4\n1950\t25009\tNewburyport\tMA\tEssex County\tH4\n1949\t25009\tMiddleton\tMA\tEssex County\tH4\n1983\t25009\tTopsfield\tMA\tEssex County\tH4\n1376\t25011\tTurners falls\tMA\tFranklin County\tH4\n1354\t25011\tGill\tMA\tFranklin County\tH4\n1351\t25011\tMontague\tMA\tFranklin County\tH4\n1330\t25011\tAshfield\tMA\tFranklin County\tH4\n1339\t25011\tCharlemont\tMA\tFranklin County\tH4\n1096\t25011\tWilliamsburg\tMA\tFranklin County\tH4\n1347\t25011\tLake pleasant\tMA\tFranklin County\tH4\n1093\t25011\tWhately\tMA\tFranklin County\tH4\n1002\t25011\tAmherst\tMA\tFranklin County\tH4\n1355\t25011\tNew salem\tMA\tFranklin County\tH4\n1375\t25011\tSunderland\tMA\tFranklin County\tH4\n1349\t25011\tMillers falls\tMA\tFranklin County\tH4\n1380\t25011\tWendell depot\tMA\tFranklin County\tH4\n1342\t25011\tDeerfield\tMA\tFranklin County\tH4\n1337\t25011\tBernardston\tMA\tFranklin County\tH4\n1340\t25011\tColrain\tMA\tFranklin County\tH4\n1039\t25011\tHaydenville\tMA\tFranklin County\tH4\n1302\t25011\tGreenfield\tMA\tFranklin County\tH4\n1247\t25011\tNorth adams\tMA\tFranklin County\tH4\n1338\t25011\tBuckland\tMA\tFranklin County\tH4\n1379\t25011\tWendell\tMA\tFranklin County\tH4\n1070\t25011\tPlainfield\tMA\tFranklin County\tH4\n1301\t25011\tGreenfield\tMA\tFranklin County\tH4\n1331\t25011\tAthol\tMA\tFranklin County\tH4\n1370\t25011\tShelburne falls\tMA\tFranklin County\tH4\n1364\t25011\tOrange\tMA\tFranklin County\tH4\n1360\t25011\tNorthfield\tMA\tFranklin County\tH4\n1072\t25011\tShutesbury\tMA\tFranklin County\tH4\n1350\t25011\tMonroe bridge\tMA\tFranklin County\tH4\n1346\t25011\tHeath\tMA\tFranklin County\tH4\n1032\t25011\tGoshen\tMA\tFranklin County\tH4\n1341\t25011\tConway\tMA\tFranklin County\tH4\n1054\t25011\tLeverett\tMA\tFranklin County\tH4\n1373\t25011\tSouth deerfield\tMA\tFranklin County\tH4\n1344\t25011\tErving\tMA\tFranklin County\tH4\n1367\t25011\tRowe\tMA\tFranklin County\tH4\n1343\t25011\tDrury\tMA\tFranklin County\tH4\n1378\t25011\tWarwick\tMA\tFranklin County\tH4\n1085\t25013\tWestfield\tMA\tHampden County\tH4\n1104\t25013\tSpringfield\tMA\tHampden County\tH4\n1103\t25013\tSpringfield\tMA\tHampden County\tH4\n1057\t25013\tMonson\tMA\tHampden County\tH4\n1095\t25013\tWilbraham\tMA\tHampden County\tH4\n1109\t25013\tSpringfield\tMA\tHampden County\tH4\n1101\t25013\tSpringfield\tMA\tHampden County\tH4\n1138\t25013\tSpringfield\tMA\tHampden County\tH4\n1199\t25013\tSpringfield\tMA\tHampden County\tH4\n1030\t25013\tFeeding hills\tMA\tHampden County\tH4\n1020\t25013\tChicopee\tMA\tHampden County\tH4\n1118\t25013\tSpringfield\tMA\tHampden County\tH4\n1071\t25013\tRussell\tMA\tHampden County\tH4\n1129\t25013\tSpringfield\tMA\tHampden County\tH4\n1022\t25013\tChicopee\tMA\tHampden County\tH4\n1079\t25013\tThorndike\tMA\tHampden County\tH4\n1014\t25013\tChicopee\tMA\tHampden County\tH4\n1069\t25013\tPalmer\tMA\tHampden County\tH4\n1073\t25013\tSouthampton\tMA\tHampden County\tH4\n1077\t25013\tSouthwick\tMA\tHampden County\tH4\n1128\t25013\tSpringfield\tMA\tHampden County\tH4\n1115\t25013\tSpringfield\tMA\tHampden County\tH4\n1111\t25013\tSpringfield\tMA\tHampden County\tH4\n1050\t25013\tHuntington\tMA\tHampden County\tH4\n1056\t25013\tLudlow\tMA\tHampden County\tH4\n1082\t25013\tWare\tMA\tHampden County\tH4\n1089\t25013\tWest springfield\tMA\tHampden County\tH4\n1107\t25013\tSpringfield\tMA\tHampden County\tH4\n1108\t25013\tSpringfield\tMA\tHampden County\tH4\n1116\t25013\tLongmeadow\tMA\tHampden County\tH4\n1223\t25013\tBecket\tMA\tHampden County\tH4\n1028\t25013\tEast longmeadow\tMA\tHampden County\tH4\n1001\t25013\tAgawam\tMA\tHampden County\tH4\n1106\t25013\tLongmeadow\tMA\tHampden County\tH4\n1119\t25013\tSpringfield\tMA\tHampden County\tH4\n1010\t25013\tBrimfield\tMA\tHampden County\tH4\n1008\t25013\tBlandford\tMA\tHampden County\tH4\n1090\t25013\tWest springfield\tMA\tHampden County\tH4\n1152\t25013\tSpringfield\tMA\tHampden County\tH4\n1097\t25013\tWoronoco\tMA\tHampden County\tH4\n1009\t25013\tBondsville\tMA\tHampden County\tH4\n1013\t25013\tChicopee\tMA\tHampden County\tH4\n1011\t25013\tChester\tMA\tHampden County\tH4\n1080\t25013\tThree rivers\tMA\tHampden County\tH4\n1040\t25013\tHolyoke\tMA\tHampden County\tH4\n1036\t25013\tHampden\tMA\tHampden County\tH4\n1521\t25013\tHolland\tMA\tHampden County\tH4\n1041\t25013\tHolyoke\tMA\tHampden County\tH4\n1021\t25013\tChicopee\tMA\tHampden County\tH4\n1033\t25013\tGranby\tMA\tHampden County\tH4\n1105\t25013\tSpringfield\tMA\tHampden County\tH4\n1151\t25013\tIndian orchard\tMA\tHampden County\tH4\n1034\t25013\tGranville\tMA\tHampden County\tH4\n1081\t25013\tWales\tMA\tHampden County\tH4\n1144\t25013\tSpringfield\tMA\tHampden County\tH4\n1139\t25013\tSpringfield\tMA\tHampden County\tH4\n1026\t25015\tCummington\tMA\tHampshire County\tH4\n1098\t25015\tWorthington\tMA\tHampshire County\tH4\n1330\t25015\tAshfield\tMA\tHampshire County\tH4\n1096\t25015\tWilliamsburg\tMA\tHampshire County\tH4\n1075\t25015\tSouth hadley\tMA\tHampshire County\tH4\n1235\t25015\tHinsdale\tMA\tHampshire County\tH4\n1003\t25015\tAmherst\tMA\tHampshire County\tH4\n1002\t25015\tAmherst\tMA\tHampshire County\tH4\n1004\t25015\tAmherst\tMA\tHampshire County\tH4\n1084\t25015\tWest chesterfield\tMA\tHampshire County\tH4\n1059\t25015\tNorth amherst\tMA\tHampshire County\tH4\n1069\t25015\tPalmer\tMA\tHampshire County\tH4\n1073\t25015\tSouthampton\tMA\tHampshire County\tH4\n1088\t25015\tWest hatfield\tMA\tHampshire County\tH4\n1039\t25015\tHaydenville\tMA\tHampshire County\tH4\n1061\t25015\tNorthampton\tMA\tHampshire County\tH4\n1050\t25015\tHuntington\tMA\tHampshire County\tH4\n1053\t25015\tLeeds\tMA\tHampshire County\tH4\n1062\t25015\tFlorence\tMA\tHampshire County\tH4\n1082\t25015\tWare\tMA\tHampshire County\tH4\n1035\t25015\tHadley\tMA\tHampshire County\tH4\n1070\t25015\tPlainfield\tMA\tHampshire 
